vi "Set Variant.vi"(8 "error in (no error)":errorcluster, 10 "Variant":variant, 11 "int32 in":refnum<class "int64.lvclass">) -> (0 "error out":errorcluster, 3 "int32 out":refnum<class "int64.lvclass">)   [LabVIEW 2020]
uses:
  int64.lvclass
  int64.lvclass/int64.ctl
  E:/Labview/LV 2020/Libs/LV Protobuf Raw/Source/Proto Type Common/Proto Type Common.lvclass
  E:/Labview/LV 2020/Libs/LV Protobuf Raw/Source/Tag/Basic Type.lvclass
  E:/Labview/LV 2020/Libs/LV Protobuf Raw/Source/Proto Value/Proto Type.lvclass
  E:/Labview/LV 2020/Libs/LV Protobuf Raw/Source/Type Serializer/Type Serializer.lvclass
  E:/Labview/LV 2020/Libs/LV Protobuf Raw/Source/String Representable/String Representable.lvclass
  E:/Labview/LV 2020/Libs/LV Protobuf Raw/Source/Wire Type Group/Wire Type Group.lvclass
  E:/Labview/LV 2020/Libs/LV Protobuf Raw/Source/Scalar Encoder/Scalar Type.lvclass
  E:/Labview/LV 2020/Libs/LV Protobuf Raw/Source/VarINT Encoder/VarINT.lvclass
  E:/Labview/LV 2020/Libs/LV Protobuf Raw/Source/int64/int64.lvclass
  Proto Type Common/Proto Type Common.lvclass
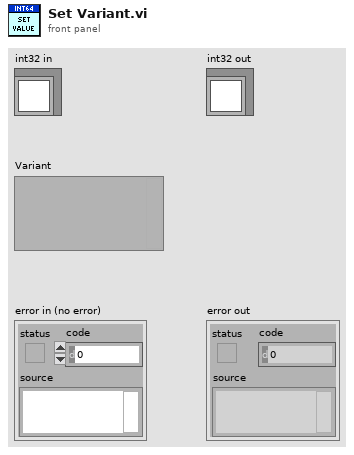
[diagram p1: front panel]
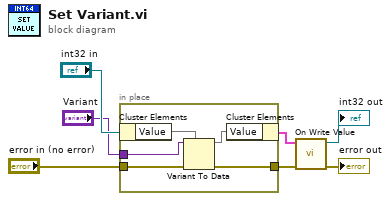
[diagram p0: block diagram]
diagram:
  n1 = in-place {
    in-place-border: "error in (no error)" -> [w12]
    in-place-border: [w11] -> w5
    in-place-border: "Variant" -> [w10]
    n2 = in-place-cluster #1("int32 in") -> ("Value"=w9)
    n3 = Variant To Data(error in=w12, type=w9, Variant=w10) -> (data=w8, error out=w11:errorcluster)
    n4 = in-place-cluster #1("Value"=w8) -> (w2:cluster{})
  }
  n5 = call "On Write Value.vi"("error in (no error)"=w5, "Proto Type Common in"=w2) -> ("error out"=→"error out":errorcluster, "Proto Type Common out"=→"int32 out":refnum<class "Proto Type Common.lvclass">)  [unwired: 8 in]
